vi "Indicate of count dives.vi"(1 "Текущий раствор":i32, 2 "Текущее погружение":i32) -> (0 "Текущее кол-во погружений в каждый стакан":i32[](array[numeric]))   [LabVIEW 2016]
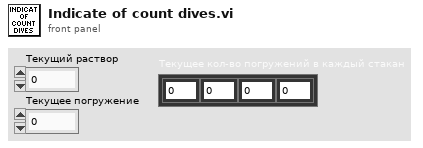
[diagram p1: front panel]
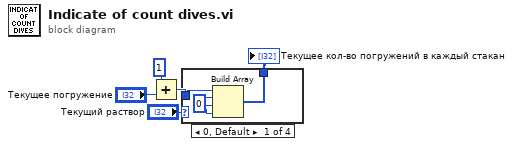
[diagram p0: block diagram]
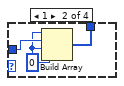
[diagram p2: hidden frame]
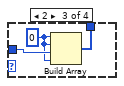
[diagram p3: hidden frame]
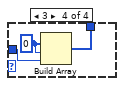
[diagram p4: hidden frame]
diagram:
  n1 = Add(x=1, y="Текущее погружение") -> (x+y=w3:i32)
  n2 = case shown="0, Default" "Текущий раствор" {
    tunnel: w3 -> [w8 w11 w14 w17]
    tunnel: [w6 w9 w12 w15] -> w4
    frame 0, Default {
      w7 = 0 ("element")
      n3 = Build Array(w8, w7, w7, w7) -> (w6:i32[])
    }
    frame 1 {
      w10 = 0 ("element")
      n4 = Build Array(w10, w11, w10, w10) -> (w9:i32[])
    }
    frame 2 {
      w13 = 0 ("element")
      n5 = Build Array(w13, w13, w14, w13) -> (w12:i32[])
    }
    frame 3 {
      w16 = 0 ("element")
      n6 = Build Array(w16, w16, w16, w17) -> (w15:i32[])
    }
  }
  "Текущее кол-во погружений в каждый стакан" <- w4
